vi "Initialize.vi"(8 "error in (no error)":errorcluster, 11 "PacificPowerSource in":refnum<class "PacificPowerSource.lvclass">) -> (0 "error out":errorcluster, 3 "PacificPowerSource out":refnum<class "PacificPowerSource.lvclass">)   [LabVIEW 2018, in "AcPwrPlugins.lvlib" / "PacificPowerSource.lvclass"]
doc: "This VI establishes communication to the instrument and optionally performs an instrument identification query and/or an instrument reset. It also places the instrument in a default state needed for other instrument driver operations. Therefore, call this VI before calling other instrument driver VIs for this instrument. Generally, you need to call the Initialize VI only once at the beginning of an application.\n\n<b>Note:</b>\nYou can clear device while you enable \"Clear Device\", and the AC power will restart."
uses:
  PacificPowerSource.lvclass
  <instrlib>/Pacific Power UPC Series/Pacific Power UPC Series.lvlib
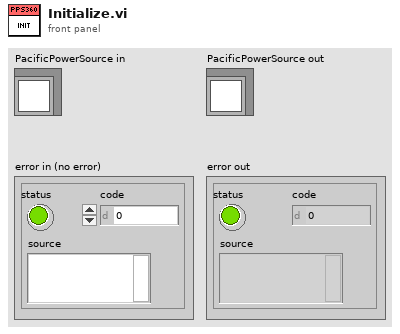
[diagram p1: front panel]
types:
  T1 = cluster{"Boolean":bool, "VISA Resource name":refnum<visa-resource-name>}[]
  T2 = typedef "AcPwrPlugins.lvlib/PacificPowerSource.lvclass/Device(s)Settings.ctl" = cluster{"MeasName":string, "Modules":cluster{"Handle":string, "Connected":bool, "Clear Device (F)":bool, "btnIdQuery":bool, "btnReset":bool, "Program #":cluster{"Phase B (Degrees)":i32, "Waveform A (1: Sine)":i32, "Voltage Level (Va)":dbl, "Program Number (0)":i32, "Voltage Level (Vb) ":dbl, "Form (3: Three)":u16, "Coupling  (0: Direct)":u16, "Frequency (45Hz)":dbl, "Current Limit (40A)":dbl, "Phase C (Degrees)":i32, "Voltage Level (Vc)":dbl, "Waveform B (1: Sine)":i32, "Waveform C (1: Sine)":i32}[], "Impedance Parameters (off, 0.00)":cluster{"State":bool, "Impedance":dbl}, "Transient Execution (F)":bool, "OutputEnabled":bool, "Source Range":cluster{"Frequency Minimum (45 Hz)":dbl, "Frequency Maximum (1200 Hz)":dbl, "Voltage Maximum (V)":dbl, "Voltage Minimum (V)":dbl, "Range Control (0: Auto)":u16, "Initial Voltage (0V)":u16, "Frequency Range (600Hz)":u16}, "Port Type":enum16{"GPIB", "Serial"}}[]}
  T3 = typedef "AcPwrPlugins.lvlib/PacificPowerSource.lvclass/Measurements.ctl" = cluster{"Handle":string, "Name":string, "Enabled ":bool, "Measurement Value":dbl, "Channel Name":enum16{"A", "B", "C"}, "Measurement Type ":T4}[]
  T4 = typedef "AcPwrPlugins.lvlib/PacificPowerSource.lvclass/MeasurementType.ctl" = enum16{"Voltage RMS L-N", "Voltage RMS L-L", "Frequency", "Current RMS", "Current Peak", "Crest Factor", "Power Factor", "Power VA", "Real Power"}
  T5 = typedef "AcPwrPlugins.lvlib/PacificPowerSource.lvclass/Modules.ctl" = cluster{"Handle":string, "Connected":bool, "Clear Device (F)":bool, "btnIdQuery":bool, "btnReset":bool, "Program #":cluster{"Phase B (Degrees)":i32, "Waveform A (1: Sine)":i32, "Voltage Level (Va)":dbl, "Program Number (0)":i32, "Voltage Level (Vb) ":dbl, "Form (3: Three)":u16, "Coupling  (0: Direct)":u16, "Frequency (45Hz)":dbl, "Current Limit (40A)":dbl, "Phase C (Degrees)":i32, "Voltage Level (Vc)":dbl, "Waveform B (1: Sine)":i32, "Waveform C (1: Sine)":i32}[], "Impedance Parameters (off, 0.00)":cluster{"State":bool, "Impedance":dbl}, "Transient Execution (F)":bool, "OutputEnabled":bool, "Source Range":cluster{"Frequency Minimum (45 Hz)":dbl, "Frequency Maximum (1200 Hz)":dbl, "Voltage Maximum (V)":dbl, "Voltage Minimum (V)":dbl, "Range Control (0: Auto)":u16, "Initial Voltage (0V)":u16, "Frequency Range (600Hz)":u16}, "Port Type":enum16{"GPIB", "Serial"}}[]
  T6 = cluster{"Handle":string, "Connected":bool, "Clear Device (F)":bool, "btnIdQuery":bool, "btnReset":bool, "Program #":cluster{"Phase B (Degrees)":i32, "Waveform A (1: Sine)":i32, "Voltage Level (Va)":dbl, "Program Number (0)":i32, "Voltage Level (Vb) ":dbl, "Form (3: Three)":u16, "Coupling  (0: Direct)":u16, "Frequency (45Hz)":dbl, "Current Limit (40A)":dbl, "Phase C (Degrees)":i32, "Voltage Level (Vc)":dbl, "Waveform B (1: Sine)":i32, "Waveform C (1: Sine)":i32}[], "Impedance Parameters (off, 0.00)":cluster{"State":bool, "Impedance":dbl}, "Transient Execution (F)":bool, "OutputEnabled":bool, "Source Range":cluster{"Frequency Minimum (45 Hz)":dbl, "Frequency Maximum (1200 Hz)":dbl, "Voltage Maximum (V)":dbl, "Voltage Minimum (V)":dbl, "Range Control (0: Auto)":u16, "Initial Voltage (0V)":u16, "Frequency Range (600Hz)":u16}, "Port Type":enum16{"GPIB", "Serial"}}
  T7 = cluster{"Handle Connected?":bool, "VISA Resource name":refnum<visa-resource-name>}
  T8 = cluster{"Handle Connected?":bool, "VISA Resource name":refnum<visa-resource-name>}[]
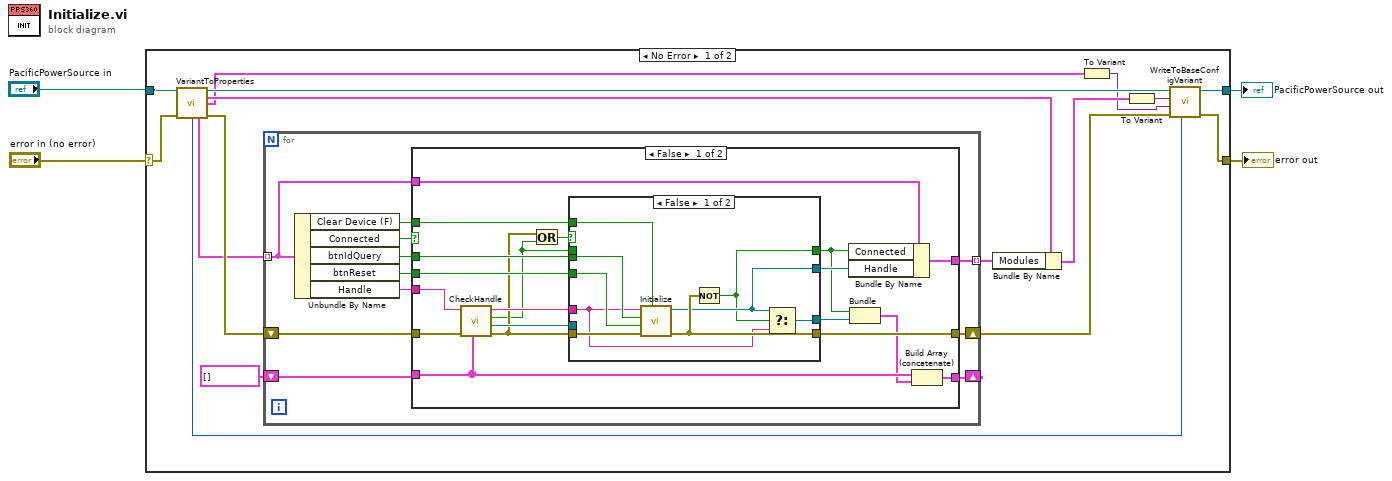
[diagram p0: block diagram]
diagram:
  n1 = case shown="No Error" "error in (no error)" {
    selector: "error in (no error)" -> [w16 w66]
    tunnel: "PacificPowerSource in" -> [w17 w67]
    tunnel: [w12 w67] -> w2
    tunnel: [w13 w66] -> w1
    frame No Error {
      n2 = call "VariantToProperties.vi"("PacificPowerSource in"=w17, "error in (no error)"=w16) -> ("PacificPowerSource out"=w11:refnum<class "PacificPowerSource.lvclass">, "Device(s)Settings"=w18:T2, "Measurements"=w6:T3, "Measurement Refresh Time (ms)"=w7:u32, "Modules"=w8:T5, "error out"=w15:errorcluster)  [unwired: 7 in, 1 out]
      n3 = for {
        shift-right: [w30] -> w14
        shift-left: w15 -> [w31]
        tunnel: w8 -> [w29] mode=indexing
        tunnel: [w28] -> w19 mode=indexing
        shift-right: [w21] -> _
        shift-left: T1 [] ("Array") -> [w22]
        n4 = Unbundle By Name(w29) -> ("Clear Device (F)"=w26:bool, "Connected"=w27:bool, "btnIdQuery"=w25:bool, "btnReset"=w24:bool, "Handle"=w23:string)
        n5 = case shown="False" w27 {
          tunnel: w31 -> [w44 w65]
          tunnel: [w46 w65] -> w30
          tunnel: w24 -> [w48 _]
          tunnel: w25 -> [w47 _]
          tunnel: w29 -> [w35 w64]
          tunnel: [w50 w64] -> w28
          tunnel: w26 -> [w45 _]
          tunnel: w23 -> [w43 _]
          tunnel: w22 -> [w37 w63]
          tunnel: [w36 w63] -> w21
          frame False {
            n6 = call "CheckHandle.vi"("Array"=w37, "Error In"=w44, "Handle In"=w43) -> ("Error Out"=w39:errorcluster, "VISA Resource name"=w40:refnum<visa-resource-name>, "Handle Connected?"=w38:bool, "Handle Out"=w42:string)  [unwired: 5 in]
            n7 = Or(x=w39, y=w38) -> (x .or. y?=w41:bool)
            n8 = case shown="False" w41 {
              tunnel: [w52 w61] -> w33
              tunnel: w39 -> [w59 w62]
              tunnel: [w54 w60] -> w49
              tunnel: w48 -> [w58 _]
              tunnel: w47 -> [w57 _]
              tunnel: [w56 w62] -> w46
              tunnel: w45 -> [w55 _]
              tunnel: w42 -> [w53 _]
              tunnel: w40 -> [_ w60]
              tunnel: w38 -> [_ w61]
              tunnel: [w51 w60] -> w34
              frame False {
                n9 = call <instrlib>:"Initialize.vi"("Clear Device (False)"=w55, "error in (no error)"=w59, "Reset (True)"=w58, "ID Query (True)"=w57, "VISA resource name"=w53) -> ("error out"=w56:errorcluster, "VISA resource name out"=w54:refnum<visa-resource-name>)  [unwired: 5 in]
                n10 = Not(x=w56) -> (.not. x?=w52:bool)
                n11 = Select(t=w54, s=w52, f=w53) -> (s? t:f=w51:refnum<visa-resource-name>)
              }
              frame True {
              }
            }
            n12 = Bundle By Name(cluster=w35, "Connected"=w33, "Handle"=w49) -> (w50:T6)
            n13 = Bundle("Handle Connected?"=w33, "VISA Resource name"=w34) -> (w32:T7)  [unwired: 1 in]
            n14 = Build Array (concatenate)(w37, w32) -> (w36:T8)
          }
          frame True {
          }
        }
      }
      n15 = Bundle By Name(cluster=w18, "Modules"=w19) -> (w9:T2)
      n16 = To Variant(anything=w6) -> (Variant=w5:variant)
      n17 = To Variant(anything=w9) -> (Variant=w10:variant)
      n18 = call "WriteToBaseConfigVariant.vi"("Measurement Refresh Time (ms)"=w7, "error in (no error)"=w14, "Meas"=w5, "Config"=w10, "PacificPowerSource in"=w11) -> ("error out"=w13:errorcluster, "PacificPowerSource out"=w12:refnum<class "PacificPowerSource.lvclass">)  [unwired: 5 in]
    }
    frame Error {
    }
  }
  "error out" <- w1
  "PacificPowerSource out" <- w2
